vi "Read & Wirte Configuration OO.vi"() -> ()   [LabVIEW 2014, in "LVOOP Introduction.lvlib"]
doc: "Read object oriented configuration data from ini-file using the configuration class.\n\nLizenziert unter EUPL V. 1.1"
uses:
  LVOOP Introduction.lvlib
  Configuration/Classes/Configuration/Configuration.lvclass
  Configuration/Classes/Ini-File/Ini-File.lvclass
  Classes/Section 1/Section 1.lvclass
  Configuration/Classes/Section/Section.lvclass
panel:
  out "Sections":T1(array[cluster])
  out "Configuration out":refnum<class "Configuration.lvclass">
  in  "Configuration File Path":path
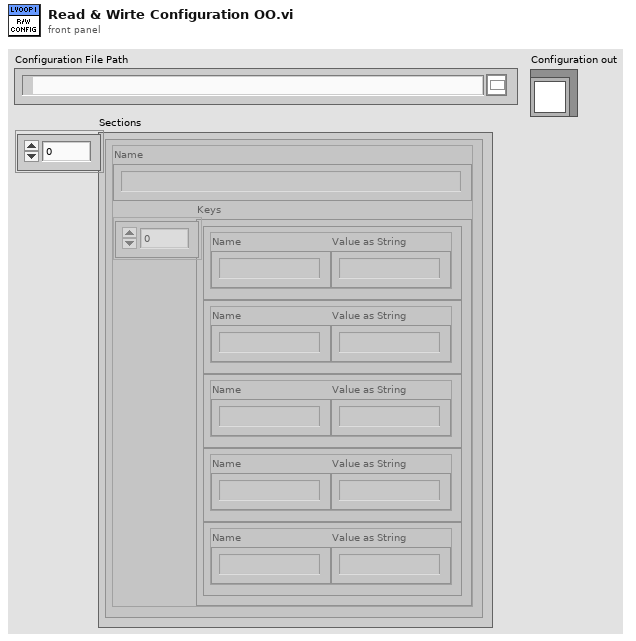
[diagram p1: front panel]
types:
  T1 = cluster{"Name":string, "Keys":cluster{"Name":string, "Value as String":string}[]}[]
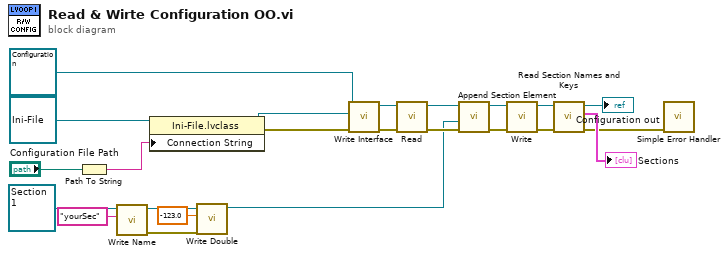
[diagram p0: block diagram]
diagram:
  n1 = Path To String(path="Configuration File Path") -> (string=w16:string)
  n2 = call "Write Name.vi"("Name"="yourSec", "Section in"=refnum<class "Section 1.lvclass"> refnum ("LVOOP Introduction.lvlib:Section 1.lvclass")) -> ("error out"=w11:errorcluster, "Section out"=w13:refnum<class "Section 1.lvclass">)  [unwired: 8 in]
  n3 = property class="Ini-File.lvclass"(reference=refnum<class "Ini-File.lvclass"> refnum ("Configuration.lvlib:Ini-File.lvclass"), "Connection String"=w16) -> (reference out=w1:refnum<class "Ini-File.lvclass">, error out=w22:errorcluster)  [unwired: 1 in]
  n4 = call "Write Double.vi"("error in (no error)"=w11, "Double"=-123.0, "Section 1 in"=w13) -> ("Section 1 out"=w8:refnum<class "Section 1.lvclass">)  [unwired: 7 in, 1 out]
  n5 = call "Write Interface.vi"("error in (no error)"=w22, "Interface"=w1, "Configuration in"=refnum<class "Configuration.lvclass"> refnum) -> ("error out"=w21:errorcluster, "Configuration out"=w20:refnum<class "Configuration.lvclass">)  [unwired: 7 in]
  n6 = call "Read.vi"("error in (no error)"=w21, "Configuration"=w20) -> ("error out"=w9:errorcluster, "Configuration out"=w10:refnum<class "Configuration.lvclass">)  [unwired: 8 in]
  n7 = call "Append Section Element.vi"("error in (no error)"=w9, "Section"=w8, "Configuration in"=w10) -> ("error out"=w6:errorcluster, "Configuration out"=w7:refnum<class "Configuration.lvclass">)  [unwired: 7 in]
  n8 = call "Write.vi"("error in (no error)"=w6, "Configuration in"=w7) -> ("error out"=w4:errorcluster, "Configuration out"=w5:refnum<class "Configuration.lvclass">)  [unwired: 8 in]
  n9 = call "Read Section Names and Keys.vi"("error in (no error)"=w4, "Configuration in"=w5) -> ("error out"=w2:errorcluster, "Sections"=→"Sections":T1, "Configuration out"=→"Configuration out":refnum<class "Configuration.lvclass">)  [unwired: 7 in]
  n10 = call <vilib>:"Simple Error Handler.vi"("error in (no error)"=w2) -> ()  [unwired: 4 in, 5 out]
